vi "_Remove Service.vi"(8 "error in (no error)":errorcluster, 10 "Type":T1, 11 "DiscoveryService in":refnum<class "NodeDiscovery.lvclass">) -> (0 "error out":errorcluster, 3 "DiscoveryService out":refnum<class "NodeDiscovery.lvclass">)   [LabVIEW 2020, in "Vecto.lvlib" / "NodeDiscovery.lvclass"]
uses:
  NodeDiscovery.lvclass
  proto/Discovery/Class/Msg.lvclass
  proto/ServiceType/Enumeration.ctl
  proto/ServiceType/ServiceType.lvlib
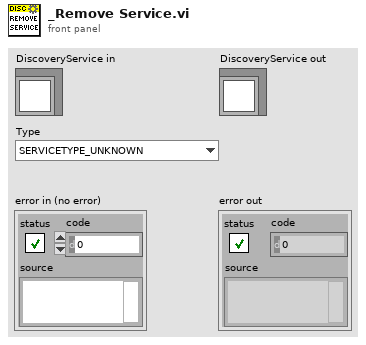
[diagram p1: front panel]
types:
  T1 = typedef "ServiceType.lvlib/Enumeration.ctl" = enum16{"SERVICETYPE_UNKNOWN", "SERVICETYPE_TCPSERVER", "SERVICETYPE_HTTPSERVER"}
  T2 = typedef "Discovery.lvlib/Data.ctl" = cluster{"node_id":u32, "name":string, "ip":u32, "status":string, "services":T3[], "system":string, "cluster":string}
  T3 = typedef "Service.lvlib/Data.ctl" = cluster{"type":T1, "port":i32}
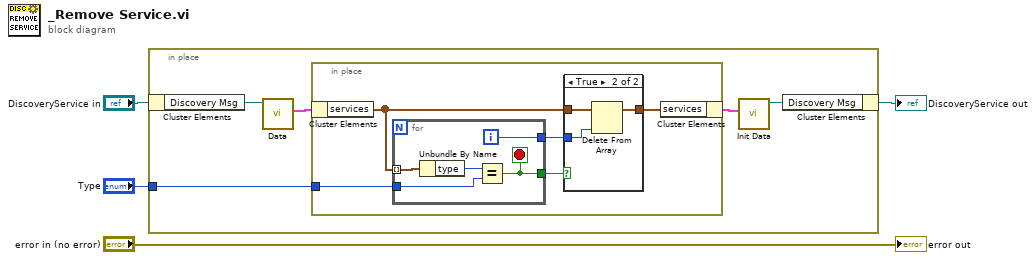
[diagram p0: block diagram]
diagram:
  n1 = in-place {
    in-place-border: "Type" -> [w5]
    n2 = in-place-cluster #1("DiscoveryService in") -> ("Discovery Msg"=w9:refnum<class "Msg.lvclass">)
    n3 = call "Data.vi"("PB Msg Template in"=w9) -> ("Data"=w8:T2)  [unwired: 8 in, 2 out]
    n4 = in-place {
      in-place-border: w5 -> [w14]
      n5 = in-place-cluster #2(w8) -> ("services"=w11:T3[])
      n6 = for {
        tunnel: w11 -> [w23] mode=indexing
        tunnel: w14 -> [w22]
        tunnel: [w20] -> w12
        tunnel: [w19] -> w13
        i -> [w20]
        stop <- w19 stop-if-true
        n7 = Unbundle By Name(w23) -> ("type"=w21:T1)
        n8 = Equal?(x=w21, y=w22) -> (x = y?=w19:bool)
      }
      n9 = case shown="True" w13 {
        tunnel: w12 -> [_ w17]
        tunnel: w11 -> [w15 w18]
        tunnel: [w15 w16] -> w10
        frame False {
        }
        frame True {
          n10 = Delete From Array(array=w18, index=w17) -> (array with subset deleted=w16:T3[])  [unwired: 1 in, 1 out]
        }
      }
      n11 = in-place-cluster #2("services"=w10) -> (w7:T2)
    }
    n12 = call "Init Data.vi"("Data"=w7) -> ("Msg out"=w6:refnum<class "Msg.lvclass">)  [unwired: 10 in]
    n13 = in-place-cluster #1("Discovery Msg"=w6) -> (→"DiscoveryService out":refnum<class "NodeDiscovery.lvclass">)
  }
  "error out" <- "error in (no error)"
